vi "Save_Scope_Image_In_PC.vi"(4 "Temp_Volt":string="Chip_L102", 5 "Base path":path, 6 "Chip":string="Chip_L102", 7 "Meas_Folder":string, 8 "error in (no error)":errorcluster, 11 "Scope_VISA":refnum<visa-resource-name>) -> (0 "error out":errorcluster, 3 "Dup VISA resource name":refnum<visa-resource-name>)   [LabVIEW 2019]
uses:
  <userlib>/_TI-LA/Instr Drivers/Oscilloscope/MSO9104A/Driver/EasyIO/Typedefs/MSO9104A Save Image Settings.ctl
  <userlib>/_TI-LA/Instr Drivers/Oscilloscope/MSO9104A/Driver/EasyIO/Typedefs/MSO9104A Image Format.ctl
  <userlib>/_TI-LA/Instr Drivers/Oscilloscope/MSO9104A/Driver/EasyIO/Typedefs/Screen Mode.ctl
  <userlib>/_TI-LA/Instr Drivers/Oscilloscope/MSO9104A/Driver/MSO9104A.lvlib
panel:
  in  "Image Settings":T1={"File Name"="Image", "Format"=enum."PNG", "Screen Mode"=enum."Screen", "Compress BMP Format? (F)"=FALSE, "Invert Image? (F)"=FALSE}
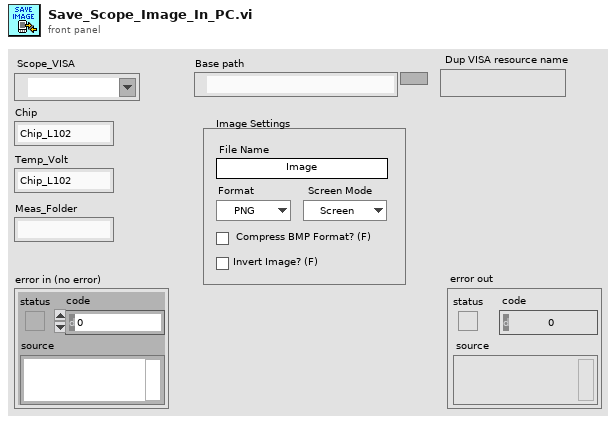
[diagram p1: front panel]
types:
  T1 = typedef "MSO9104A.lvlib/MSO9104A Save Image Settings.ctl" = cluster{"File Name":string, "Format":T2, "Screen Mode":T3, "Compress BMP Format? (F)":bool, "Invert Image? (F)":bool}
  T2 = typedef "MSO9104A.lvlib/MSO9104A Image Format.ctl" = enum16{"BMP", "GIF", "TIF", "JPEG", "PNG"}
  T3 = typedef "MSO9104A.lvlib/Screen Mode.ctl" = enum16{"Screen", "Graticule"}
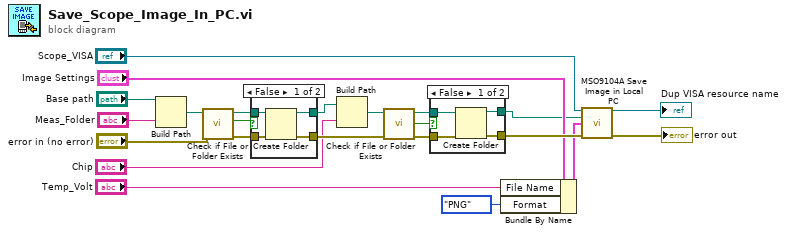
[diagram p0: block diagram]
diagram:
  n1 = Build Path(base path="Base path", name or relative path="Meas_Folder") -> (appended path=w16:path)
  n2 = call <vilib>:"Check if File or Folder Exists.vi"("error in (no error)"="error in (no error)", "path"=w16) -> ("error out"=w22:errorcluster, "file or folder exists?"=w23:bool, "dup path"=w21:path)  [unwired: 7 in]
  n3 = case shown="False" w23 {
    tunnel: w22 -> [w27 w28]
    tunnel: w21 -> [w26 w29]
    tunnel: [w25 w28] -> w20
    tunnel: [w24 w29] -> w12
    frame False {
      n4 = Create Folder(path (use dialog)=w26, error in=w27) -> (created path=w24:path, error out=w25:errorcluster)  [unwired: 1 in, 1 out]
    }
    frame True {
    }
  }
  n5 = Build Path(base path=w12, name or relative path="Chip") -> (appended path=w13:path)
  n6 = call <vilib>:"Check if File or Folder Exists.vi"("error in (no error)"=w20, "path"=w13) -> ("error out"=w19:errorcluster, "file or folder exists?"=w17:bool, "dup path"=w18:path)  [unwired: 7 in]
  n7 = case shown="False" w17 {
    tunnel: w19 -> [w33 w34]
    tunnel: w18 -> [w32 w35]
    tunnel: [w31 w34] -> w9
    tunnel: [w30 w35] -> w3
    frame False {
      n8 = Create Folder(path (use dialog)=w32, error in=w33) -> (created path=w30:path, error out=w31:errorcluster)  [unwired: 1 in, 1 out]
    }
    frame True {
    }
  }
  n9 = Bundle By Name(cluster="Image Settings", "File Name"="Temp_Volt", "Format"=MSO9104A_Image_Format."PNG") -> (w5:T1)
  n10 = call <userlib>:"MSO9104A Save Image in Local PC.vi"("VISA resource name"="Scope_VISA", "Save Folder Path"=w3, "Image Settings"=w5, "error in"=w9) -> ("Dup VISA resource name"=→"Dup VISA resource name":refnum<visa-resource-name>, "error out"=→"error out":errorcluster)  [unwired: 9 in, 1 out]
